vi "Equal.vi"(1 "Y":variant, 2 "X":variant) -> (0 "Equal?":bool)   [LabVIEW 2019, in "UnitTestFramework.lvclass"]
uses:
  UT/UnitTestFramework.lvclass
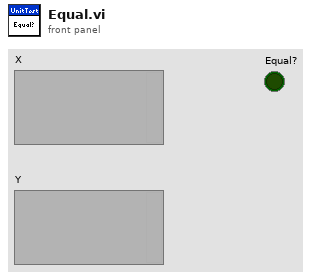
[diagram p1: front panel]
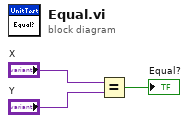
[diagram p0: block diagram]
diagram:
  n1 = Equal?(x="X", y="Y") -> (x = y?=→"Equal?":bool)
